vi "AE ListBox.vi"(7 "Action":T1(ring), 8 "error in (no error)":errorcluster, 9 "input pressure":dbl, 11 "input listbox":cluster{"CtlRef":refnum<vi>, "Row":i32}) -> (0 "error out":errorcluster, 1 "output pressure":dbl, 3 "output listbox":cluster{"CtlRef":refnum<vi>, "Row":i32})   [LabVIEW 2013, in "main.lvlib"]
uses:
  main.lvlib
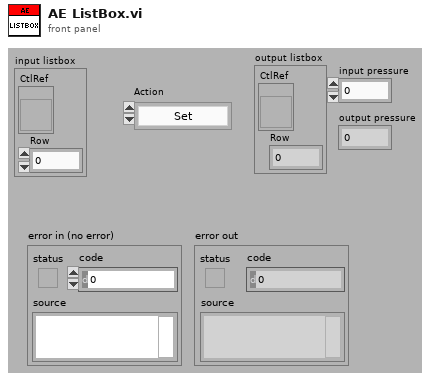
[diagram p1: front panel]
types:
  T1 = enum16{"Set", "Init", "Get Pressure", "Set Pressure", "Get"}
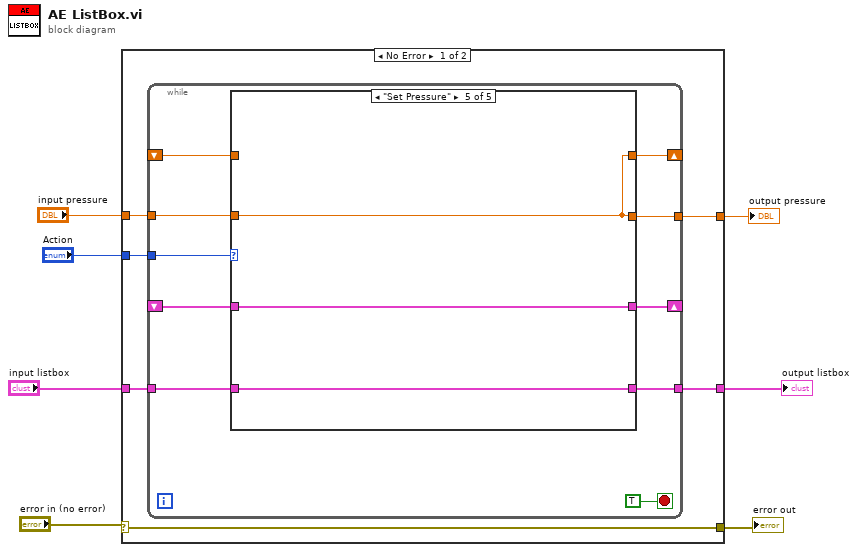
[diagram p0: block diagram]
diagram:
  n1 = case shown="No Error" "error in (no error)" {
    selector: "error in (no error)" -> [w10 w41]
    tunnel: "Action" -> [w13 _]
    tunnel: "input listbox" -> [w12 w40]
    tunnel: [w11 w40] -> w5
    tunnel: [w10 w41] -> w3
    tunnel: [w9 w39] -> w2
    tunnel: "input pressure" -> [w8 w39]
    frame No Error {
      n2 = while {
        shift-right: [w21] -> _
        shift-left: _ -> [w20]
        tunnel: w13 -> [w23]
        tunnel: w12 -> [w22]
        tunnel: [w19] -> w11
        shift-right: [w17] -> _
        shift-left: _ -> [w16]
        tunnel: [w15] -> w9
        tunnel: w8 -> [w14]
        stop <- TRUE stop-if-true
        n3 = case shown="\"Set Pressure\"" w23 {
          tunnel: w22 -> [w26 _ _ w33 w36]
          tunnel: [w26 w29 w32 w35 w37] -> w21
          tunnel: w20 -> [_ w29 w32 w35 w37]
          tunnel: [w26 w29 w32 w33 w36] -> w19
          tunnel: [w25 w27 w31 w34 w38] -> w17
          tunnel: w16 -> [w25 w27 w31 w34 _]
          tunnel: [w24 w28 w30 w34 w38] -> w15
          tunnel: w14 -> [w24 w28 w30 _ w38]
          frame "Set" {
          }
          frame "Init", Default {
          }
          frame "Get" {
          }
          frame "Get Pressure" {
          }
          frame "Set Pressure" {
          }
        }
      }
    }
    frame Error {
    }
  }
  "output listbox" <- w5
  "error out" <- w3
  "output pressure" <- w2
